vi "Check_Measurement_Setups.vi"(0 "Measurement Setup String":string) -> (1 "Measurement Setup String Out":string, 2 "Error Comments":string)   [LabVIEW 2010]
uses:
  File/Setup_Filetype.ctl
  Globals/Trav_pos_global.vi
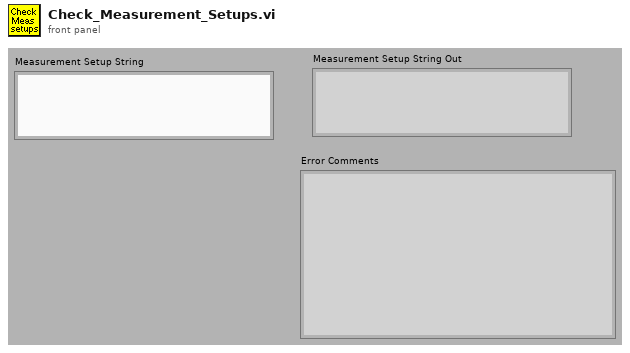
[diagram p1: front panel]
types:
  T1 = typedef "Setup_Filetype.ctl" = enum16{"Measurement Setups", "Calibration Setups", "General", "Results File Plotter Setups", "Speed Calib Tweaks"}
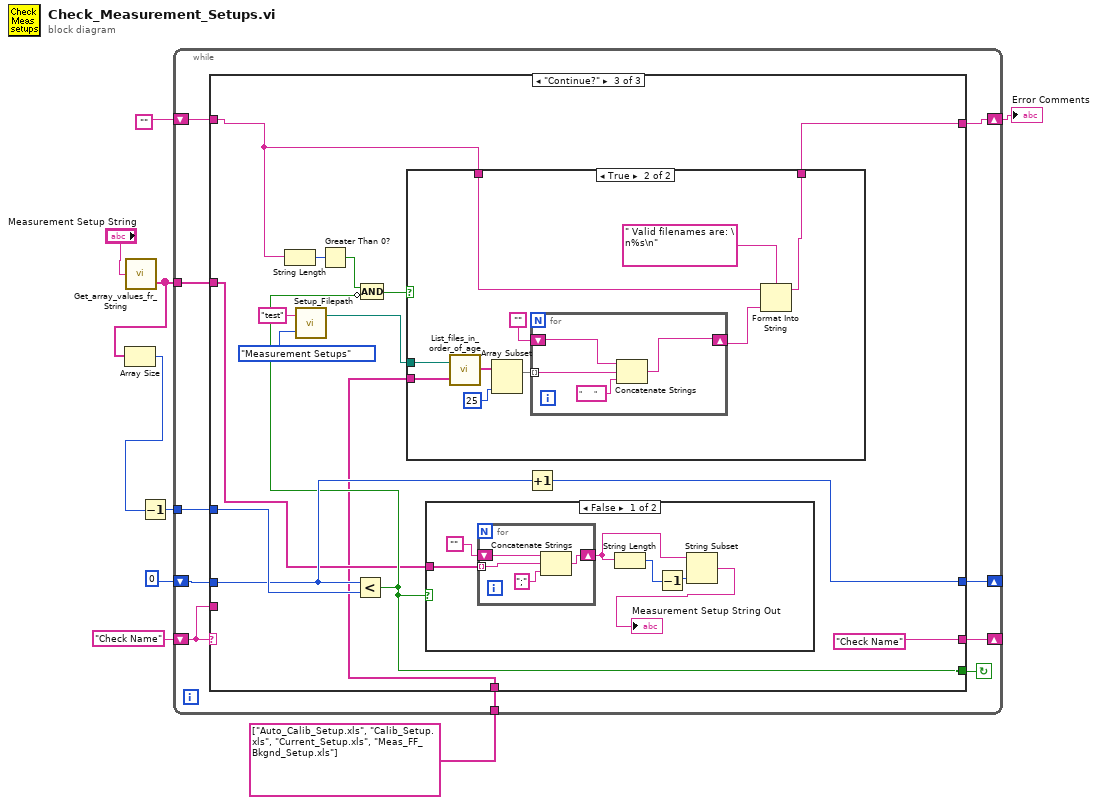
[diagram p0: block diagram]
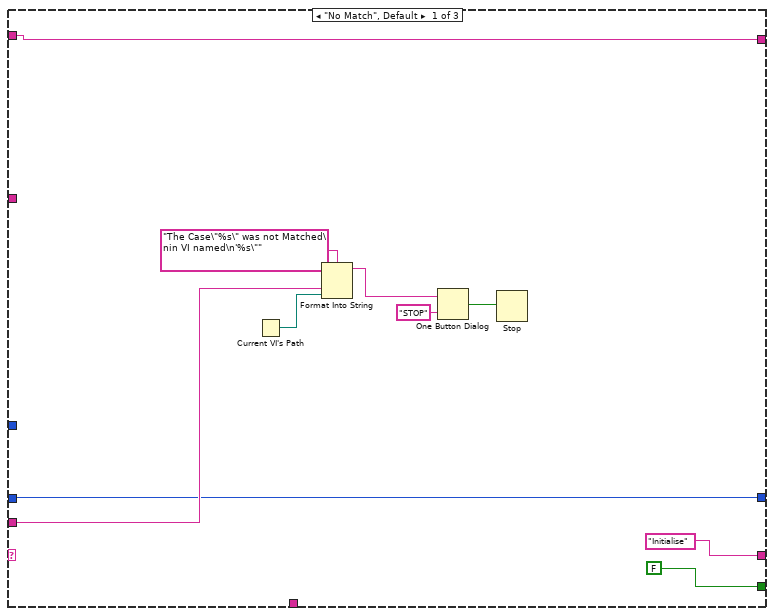
[diagram p2: hidden frame]
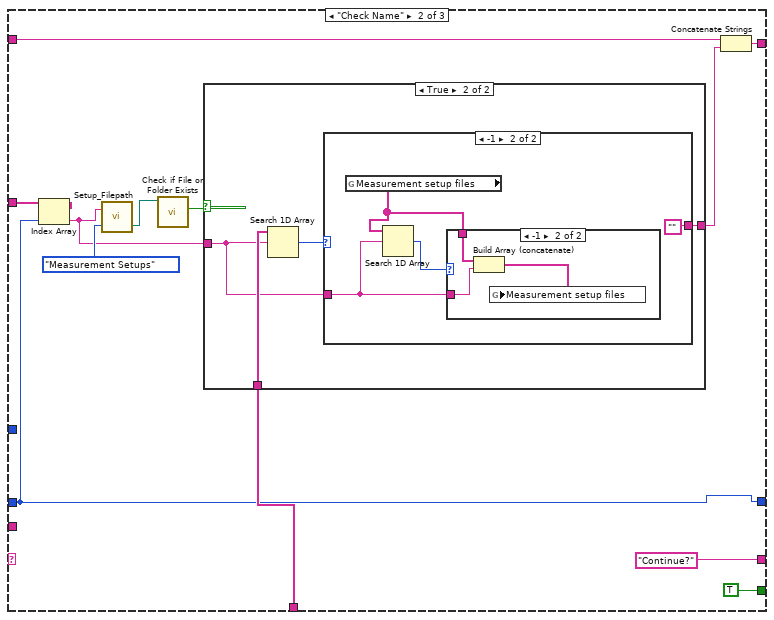
[diagram p3: hidden frame]
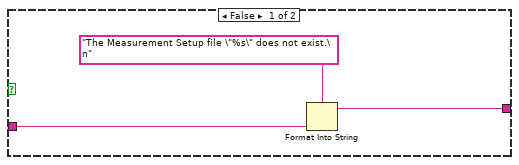
[diagram p4: hidden frame]
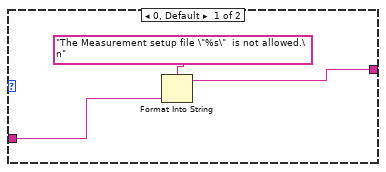
[diagram p5: hidden frame]
diagram:
  n1 = call "Get_array_values_fr_String.vi"("String Value"="Measurement Setup String") -> ("String array"=w6:string[])  [unwired: 1 out]
  n2 = Array Size(array=w6) -> (size(s)=w5:i32)
  n3 = Decrement(x=w5) -> (x-1=w4:i32)
  n4 = while {
    shift-left: "Check Name" -> [w17]
    shift-right: [w18] -> _
    shift-right: [w13] -> _
    shift-left: 0 -> [w16]
    tunnel: w6 -> [w15]
    tunnel: w4 -> [w14]
    shift-right: [w12] -> w1
    shift-left: "" -> [w11]
    tunnel: string[] ["Auto_Calib_Setup.xls", "Calib_Setup.xls", "Current_Setup.xls", "Meas_FF_Bkgnd_Setup.xls"] ("file names") -> [w10]
    stop <- w19 continue-if-true
    n5 = case shown="\"Continue?\"" w17 {
      tunnel: [FALSE TRUE w64] -> w19
      tunnel: ["Initialise" "Continue?" "Check Name"] -> w18
      tunnel: w17 -> [w24 _ _]
      tunnel: w16 -> [w21 w33 w72]
      tunnel: w15 -> [_ w41 w63]
      tunnel: w14 -> [_ _ w73]
      tunnel: [w21 w33 w71] -> w13
      tunnel: [w20 w39 w65] -> w12
      tunnel: w11 -> [w20 w37 w66]
      tunnel: w10 -> [_ w34 w62]
      frame "No Match", Default {
        n6 = Current VI's Path() -> (path=w23:path)
        n7 = Format Into String(format string="The Case\"%s\" was not Matched\nin VI named\n'%s\"" ("Format String"), w24, w23) -> (resulting string=w27:string)  [unwired: 2 in, 1 out]
        n8 = One Button Dialog(message=w27, button name ("OK")="STOP") -> (true=w25:bool)
        n9 = Stop(stop? (T)=w25) -> ()
      }
      frame "Check Name" {
        n10 = Index Array(array=w41, index=w33) -> (element=w31:string)
        n11 = call "Setup_Filepath.vi"("Setup File Type"=Setup_Filetype."Measurement Setups", "Filename in"=w31) -> ("Filename Out"=w30:path)  [unwired: 1 out]
        n12 = call <vilib>:"Check if File or Folder Exists.vi"("path"=w30) -> ("file or folder exists?"=w40:bool)  [unwired: 1 in, 9 out]
        n13 = case shown="True" w40 {
          tunnel: w31 -> [w43 w45]
          tunnel: [w42 w46] -> w38
          tunnel: w34 -> [_ w48]
          frame False {
            n14 = Format Into String(format string="The Measurement Setup file \"%s\" does not exist.\n" ("Format String"), w43) -> (resulting string=w42:string)  [unwired: 2 in, 1 out]
          }
          frame True {
            n15 = Search 1D Array(1D array=w48, element=w45) -> (index of element=w47:i32)  [unwired: 1 out]
            n16 = case shown="-1" w47 {
              tunnel: [w50 ""] -> w46
              tunnel: w45 -> [w49 w53]
              frame 0, Default {
                n17 = Format Into String(format string="The Measurement setup file \"%s\"  is not allowed.\n" ("f"), w49) -> (resulting string=w50:string)  [unwired: 2 in, 1 out]
              }
              frame -1 {
                n18 = global read "Trav_pos_global.vi" "Measurement setup files"() -> (w54:string[])
                n19 = Search 1D Array(1D array=w54, element=w53) -> (index of element=w55:i32)  [unwired: 1 out]
                n20 = case shown="-1" w55 {
                  tunnel: w54 -> [_ w58]
                  tunnel: w53 -> [_ w57]
                  frame 0, Default {
                  }
                  frame -1 {
                    n21 = Build Array (concatenate)(w58, w57) -> (w56:string[])
                    n22 = global write "Trav_pos_global.vi" "Measurement setup files"(w56) -> ()
                  }
                }
              }
            }
          }
        }
        n23 = Concatenate Strings(w37, w38) -> (w39:string)
      }
      frame "Continue?" {
        n24 = String Length(string=w66) -> (length=w69:i32)
        n25 = call "Setup_Filepath.vi"("Setup File Type"=Setup_Filetype."Measurement Setups", "Filename in"="test") -> ("Directory"=w60:path)  [unwired: 1 out]
        n26 = Greater Than 0?(x=w69) -> (x > 0?=w68:bool)
        n27 = Less?(x=w72, y=w73) -> (x < y?=w64:bool)
        n28 = Compound Arithmetic op=AND(w68, invert w64) -> (w67:bool)
        n29 = case shown="True" w67 {
          tunnel: w66 -> [w84 w88]
          tunnel: [w84 w87] -> w65
          tunnel: w62 -> [_ w86]
          tunnel: w60 -> [_ w85]
          frame False {
          }
          frame True {
            n30 = call "List_files_in_order_of_age.vi"("Files to Hide"=w86, "Folder"=w85) -> ("file names"=w90:string[])
            n31 = Array Subset(array=w90, length=25 ("Array Length")) -> (w92:string[])  [unwired: 1 in]
            n32 = for {
              shift-right: [w97] -> w94
              shift-left: "" -> [w98]
              tunnel: w92 -> [w96] mode=indexing
              n33 = Concatenate Strings(w98, w96, "      " ("Substring")) -> (w97:string)
            }
            n34 = Format Into String(format string=" Valid filenames are: \n%s\n" ("Format String"), initial string=w88, w94) -> (resulting string=w87:string)  [unwired: 1 in, 1 out]
          }
        }
        n35 = case shown="False" w64 {
          tunnel: w63 -> [w79 _]
          frame False {
            n36 = for {
              shift-right: [w80] -> w76
              shift-left: "" -> [w83]
              tunnel: w79 -> [w82] mode=indexing
              n37 = Concatenate Strings(w83, w82, ";") -> (w80:string)
            }
            n38 = String Length(string=w76) -> (length=w77:i32)
            n39 = Decrement(x=w77) -> (x-1=w75:i32)
            n40 = String Subset(string=w76, length (rest)=w75) -> (substring=→"Measurement Setup String Out":string)  [unwired: 1 out]
          }
          frame True {
          }
        }
        n41 = Increment(x=w72) -> (x+1=w71:i32)
      }
    }
  }
  "Error Comments" <- w1
